vi "calcAddressInMemory.vi"(0 "Width":u16, 1 "Rows":u16, 3 "delayRowCount":u16, 5 "Cols":u16, 8 "divider":u8) -> (7 "addressInMemory":u16)   [LabVIEW 2016]
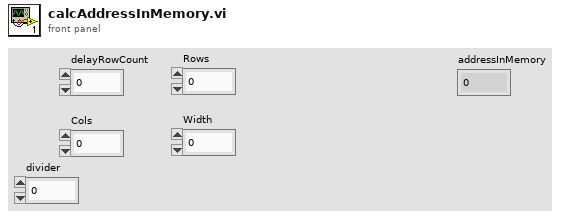
[diagram p1: front panel]
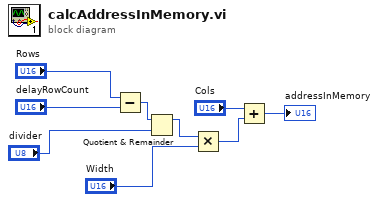
[diagram p0: block diagram]
diagram:
  n1 = Subtract(x="Rows", y="delayRowCount") -> (x-y=w4:u16)
  n2 = Quotient & Remainder(x=w4, y="divider") -> (x-y*floor(x/y)=w5:u16)  [unwired: 1 out]
  n3 = Multiply(x=w5, y="Width") -> (x*y=w6:u16)
  n4 = Add(x="Cols", y=w6) -> (x+y=→"addressInMemory":u16)
